vi "Demo Trigger.vi"(2 "Waveform 2 In":dbl[](array[numeric]) format="%.2f", 3 "Waveform 1 In":dbl[](array[numeric]) format="%.2f", 5 "Source":bool, 6 "Slope":bool, 7 "Level":dbl format="%.2f") -> (0 "Waveform 2 Out":dbl[](array[numeric]) format="%.2f", 1 "Waveform 1 Out":dbl[](array[numeric]) format="%.2f")   [LabVIEW 2009]
panel:
  # "Pos\nNeg"
  # "CH B\nEXT"
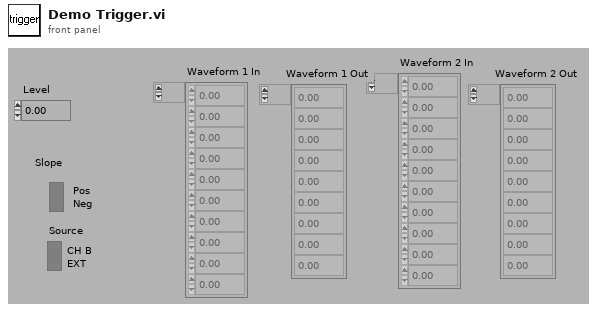
[diagram p1: front panel]
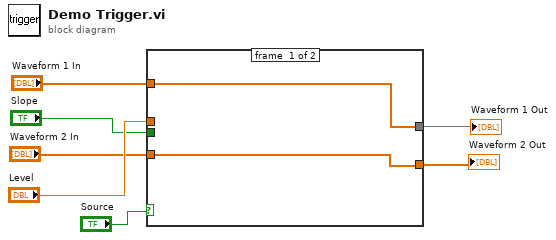
[diagram p0: block diagram]
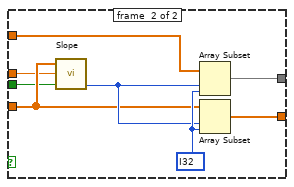
[diagram p2: hidden frame]
diagram:
  n1 = case shown="True" "Source" {
    tunnel: [w8 w17] -> w3
    tunnel: [w9 w16] -> w4
    tunnel: "Waveform 2 In" -> [w8 w13]
    tunnel: "Slope" -> [_ w12]
    tunnel: "Level" -> [_ w11]
    tunnel: "Waveform 1 In" -> [w9 w10]
    frame #0 {
    }
    frame #1 {
      w15 = i32 ?
      n2 = call "Slope.vi"("direction"=w12, "level"=w11, "array"=w13) -> ("index"=w14:i32)
      n3 = Array Subset(array=w10, index=w14, length=w15) -> (w16:dbl[])
      n4 = Array Subset(array=w13, index=w14, length=w15) -> (w17:dbl[])
    }
  }
  "Waveform 1 Out" <- w4
  "Waveform 2 Out" <- w3
